vi "Populate SCL.vi"(8 "error in":errorcluster, 11 "SCL":refnum<vi>) -> (0 "error out":errorcluster, 3 "At least one template file found?":bool)   [LabVIEW 2021]
doc: "Populates the SCL that displays the available VI templates and CTL templates, respectively.\n\nSCL = Single-Column Listbox"
uses:
  <vilib>/Utility/miscctls.llb/LVFontTypeDef.ctl
panel:
  out "All Template Filenames":string[](array[string])
  out "CTTs":string[](array[string])
  out "VITs":string[](array[string])
  out "VIs":string[](array[string])
  out "CTLs":string[](array[string])
  out "Templates Folder Location":path
  out "All Filenames In Folder":string[](array[string])
  # "Development\ncontrols/indicators useful for development and testing, but which are not outputs of the VI"
  # "Input\nInputs to the VI"
  # "Output\nOutputs of the VI"
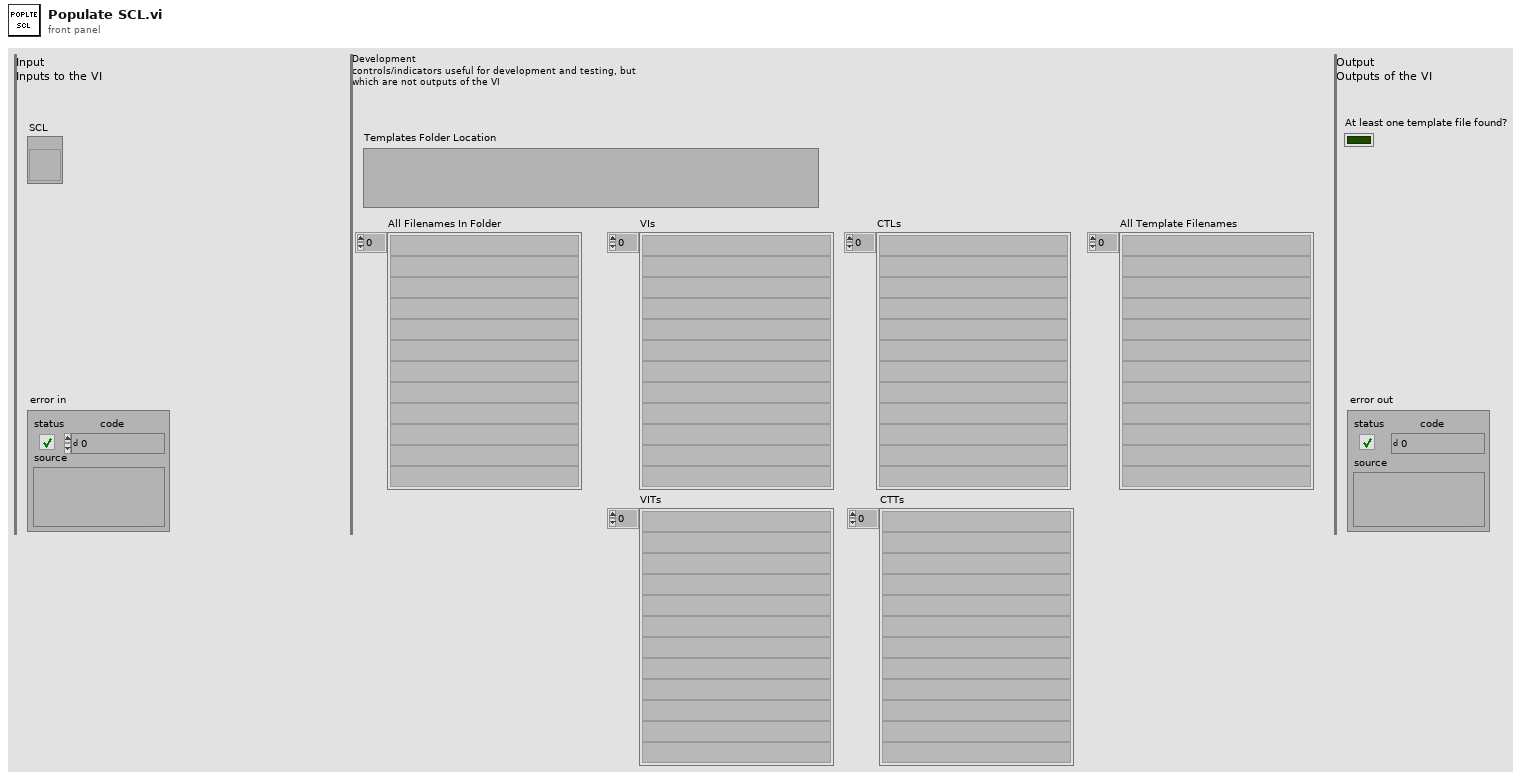
[diagram p1: front panel]
types:
  T1 = typedef "LVFontTypeDef.ctl" = cluster{"Font Name":string, "Size":u16, "Bold":bool, "Italic":bool, "Underline":bool, "Strikeout":bool, "Color":u32}
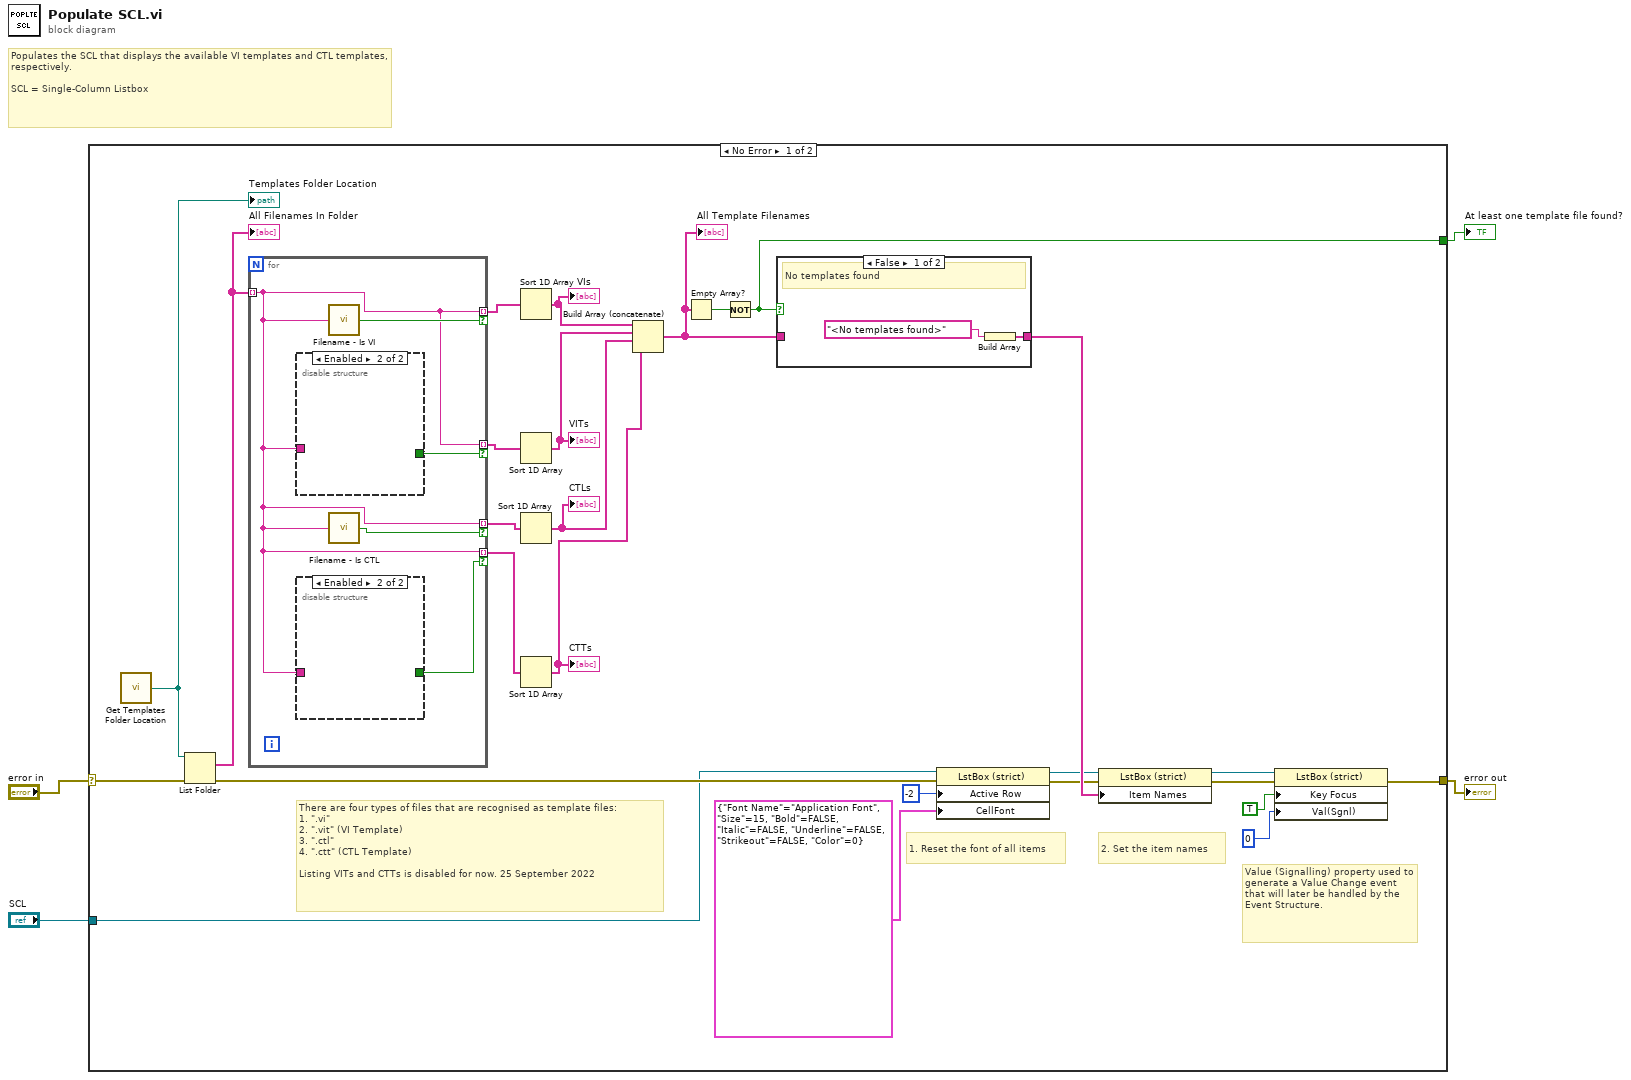
[diagram p0: block diagram]
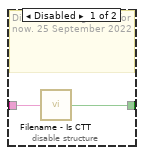
[diagram p3: hidden frame]
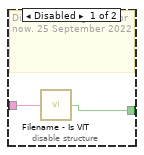
[diagram p4: hidden frame]
diagram:
  # "Populates the SCL that displays the available VI templates and CTL templates, respectively.\n\nSCL = Single-Column Listbox"
  n1 = case shown="No Error" "error in" {
    selector: "error in" -> [w30 w43]
    tunnel: [w22 w43] -> w3
    tunnel: "SCL" -> [w26 _]
    tunnel: [w6 _] -> w1
    frame No Error {
      # "Value (Signalling) property used to generate a Value Change event that will later be handled by the Event Structure."
      # "2. Set the item names"
      # "1. Reset the font of all items"
      # "There are four types of files that are recognised as template files:\n1. \".vi\"\n2. \".vit\" (VI Template)\n3. \".ctl\"\n4. \".ctt\" (CTL Template)\n\nListing VITs and CTTs is disabled for now. 25 September 2022"
      n2 = call "Get Templates Folder Location.vi"() -> ("Templates Folder Location"=w23:path)
      "Templates Folder Location" <- w23
      n3 = List Folder(path=w23, error in=w30) -> (filenames=w28:string[], error out=w29:errorcluster)  [unwired: 2 in, 2 out]
      "All Filenames In Folder" <- w28
      n4 = for {
        tunnel: w28 -> [w35] mode=indexing
        tunnel: [w35] -> w27 mode=indexing if=w38
        tunnel: [w35] -> w19 mode=indexing if=w37
        tunnel: [w35] -> w18 mode=indexing if=w36
        tunnel: [w35] -> w17 mode=indexing if=w34
        n5 = disable-structure shown="Enabled" {
          disable-tunnel: [w42 _] -> w37
          disable-tunnel: w35 -> [w41 _]
          frame Disabled {
            # "Disabled listing VIT's for now. 25 September 2022"
            n6 = call "Filename - Is VIT.vi"("Filename (including file extension)"=w41) -> ("Is VIT?"=w42:bool)
          }
          frame Enabled {
          }
        }
        n7 = disable-structure shown="Enabled" {
          disable-tunnel: w35 -> [w40 _]
          disable-tunnel: [w39 _] -> w34
          frame Disabled {
            # "Disabled listing CTT's for now. 25 September 2022"
            n8 = call "Filename - Is CTT.vi"("Filename (including file extension)"=w40) -> ("Is CTT?"=w39:bool)
          }
          frame Enabled {
          }
        }
        n9 = call "Filename - Is VI.vi"("Filename (including file extension)"=w35) -> ("Is VI?"=w38:bool)
        n10 = call "Filename - Is CTL.vi"("Filename (including file extension)"=w35) -> ("Is CTL?"=w36:bool)
      }
      n11 = Sort 1D Array(array=w27) -> (sorted array=w16:string[])
      "VIs" <- w16
      n12 = Sort 1D Array(array=w19) -> (sorted array=w15:string[])
      "VITs" <- w15
      n13 = Sort 1D Array(array=w18) -> (sorted array=w14:string[])
      "CTLs" <- w14
      n14 = Sort 1D Array(array=w17) -> (sorted array=w13:string[])
      "CTTs" <- w13
      n15 = Build Array (concatenate)(w16, w15, w14, w13) -> (w7:string[])
      "All Template Filenames" <- w7
      n16 = Empty Array?(array=w7) -> (empty?=w25:bool)
      n17 = Not(x=w25) -> (.not. x?=w6:bool)
      n18 = case shown="False" w6 {
        tunnel: w7 -> [_ w33]
        tunnel: [w31 w33] -> w12
        frame False {
          # "No templates found"
          n19 = Build Array("<No templates found>") -> (w31:string[])
        }
        frame True {
          # "One or more template files found"
        }
      }
      n20 = property class="LstBox (strict)"(reference=w26, error in=w29, "Active Row"=-2 ("Active Row:Active Row Number"), "CellFont"=T1 {"Font Name"="Application Font", "Size"=15, "Bold"=FALSE, "Italic"=FALSE, "Underline"=FALSE, "Strikeout"=FALSE, "Color"=0} ("Active Row:Cell Font")) -> (reference out=w10:refnum<vi>, error out=w9:errorcluster)
      n21 = property class="LstBox (strict)"(reference=w10, error in=w9, "Item Names"=w12) -> (reference out=w21:refnum<vi>, error out=w24:errorcluster)
      n22 = property class="LstBox (strict)"(reference=w21, error in=w24, "Key Focus"=TRUE, "Val(Sgnl)"=0 ("Value (Signaling)")) -> (error out=w22:errorcluster)  [unwired: 1 out]
    }
    frame Error {
    }
  }
  "error out" <- w3
  "At least one template file found?" <- w1
